vi "Check Mode.vi"(8 "error in (no error)":errorcluster, 11 "RT Data in in":T1 {"Channels"."Voltage"."Ref"."Data Reference" format="%.0x"; "Channels"."Current"."Ref"."Data Reference" format="%.0x"; "Channels"."Read Volt"."Ref" format="%.0x"; "Channels"."Mode"."Ref" format="%.0x"}) -> (0 "error out":errorcluster, 3 "RT Data out":T1 {"Channels"."Voltage"."Ref"."Data Reference" format="%.0x"; "Channels"."Current"."Ref"."Data Reference" format="%.0x"; "Channels"."Read Volt"."Ref" format="%.0x"; "Channels"."Mode"."Ref" format="%.0x"})   [LabVIEW 2011, in "Switch-DMM Custom Device.lvlib"]
uses:
  Switch-DMM Custom Device.lvlib
  Controls/RT Data.ctl
  Controls/Channels.ctl
  Controls/Single Channel.ctl
  <vilib>/NI Veristand/Custom Device API/Data Reference.ctl
  Controls/Block Channels.ctl
  <vilib>/NI Veristand/Custom Device API/Block Data Reference.ctl
  Controls/Communication.ctl
  Controls/Async Status.ctl
  Controls/Async State.ctl
  Controls/Async Command.ctl
  Controls/Async Events.ctl
  <vilib>/NI Veristand/Custom Device API/Global Data Refs.vi
  <vilib>/NI Veristand/Custom Device API/Custom Device API.lvlib
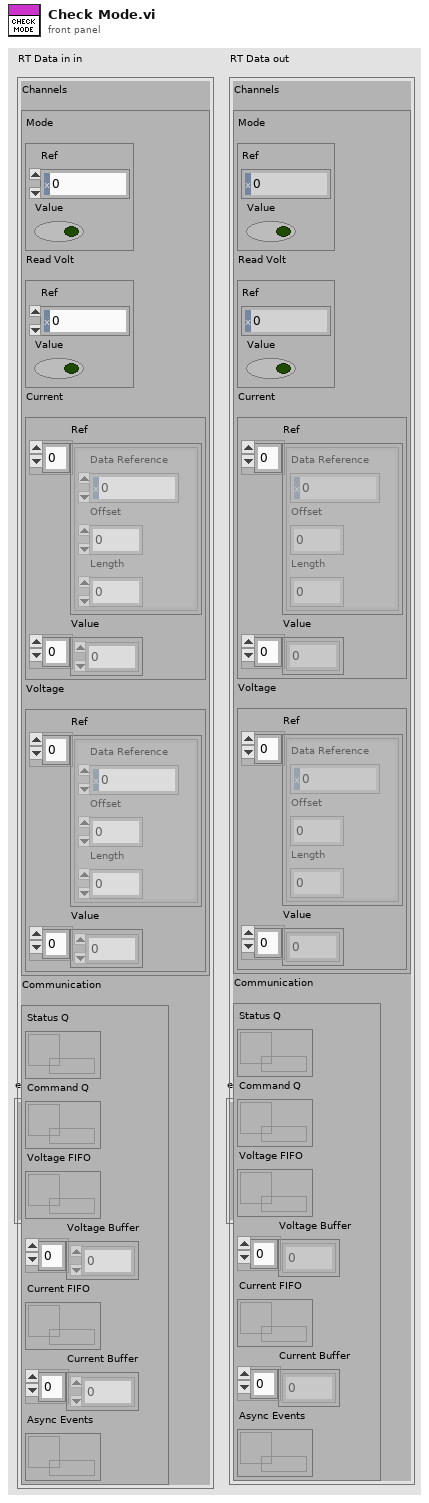
[diagram p1: front panel]
types:
  T1 = typedef "Switch-DMM Custom Device.lvlib/RT Data.ctl" = cluster{"Channels":T2, "Communication":T7}
  T2 = typedef "Switch-DMM Custom Device.lvlib/Channels.ctl" = cluster{"Mode":T3, "Read Volt":T3, "Current":T5, "Voltage":T5}
  T3 = typedef "Switch-DMM Custom Device.lvlib/Single Channel.ctl" = cluster{"Ref":T4, "Value":bool}
  T4 = typedef "Custom Device API.lvlib/Data Reference.ctl" = i32
  T5 = typedef "Switch-DMM Custom Device.lvlib/Block Channels.ctl" = cluster{"Ref":T6[], "Value":dbl[]}
  T6 = typedef "Custom Device API.lvlib/Block Data Reference.ctl" = cluster{"Data Reference":T4, "Offset":i32, "Length":i32}
  T7 = typedef "Switch-DMM Custom Device.lvlib/Communication.ctl" = cluster{"Status Q":refnum<queue>, "Command Q":refnum<queue>, "Voltage FIFO":refnum<k33>, "Voltage Buffer":dbl[], "Current FIFO":refnum<k33>, "Current Buffer":dbl[], "Async Events":refnum<queue>}
  T8 = typedef "Switch-DMM Custom Device.lvlib/Async Command.ctl" = enum16{"None", "Start", "Set Cur Mode", "Req Volt Mode", "Set Volt Mode", "Read Volt", "Exit"}
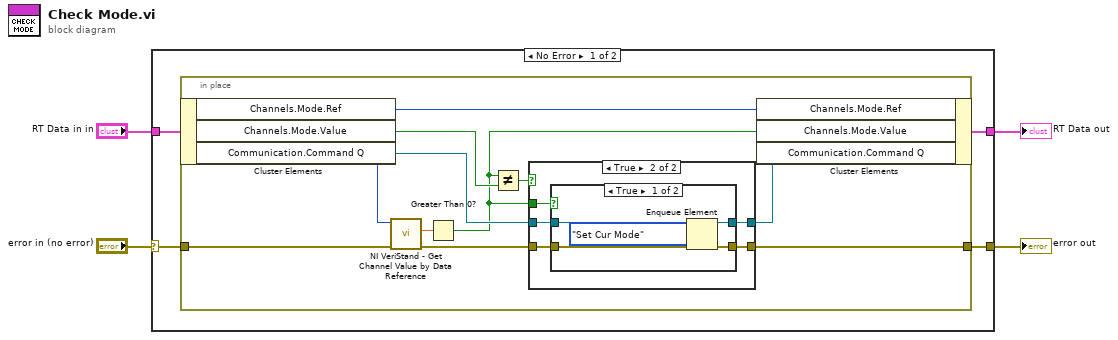
[diagram p0: block diagram]
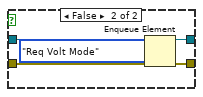
[diagram p3: hidden frame]
diagram:
  n1 = case shown="No Error" "error in (no error)" {
    selector: "error in (no error)" -> [w8 w36]
    tunnel: "RT Data in in" -> [w7 w37]
    tunnel: [w6 w37] -> w3
    tunnel: [w5 w36] -> w4
    frame No Error {
      n2 = in-place {
        in-place-border: w8 -> [w17]
        in-place-border: [w10] -> w5
        n3 = in-place-cluster #1(w7) -> ("Channels.Mode.Ref"=w18:T4, "Channels.Mode.Value"=w16:bool, "Communication.Command Q"=w13:refnum<queue>)
        n4 = call <vilib>:"NI VeriStand - Get Channel Value by Data Reference.vi"("error in (no error)"=w17, "Data Reference in"=w18) -> ("error out"=w11:errorcluster, "Value"=w14:dbl)  [unwired: 8 in]
        n5 = Greater Than 0?(x=w14) -> (x > 0?=w9:bool)
        n6 = Not Equal?(x=w9, y=w16) -> (x != y?=w15:bool)
        n7 = case shown="True" w15 {
          tunnel: w13 -> [w20 w24]
          tunnel: w9 -> [_ w25]
          tunnel: [w20 w23] -> w12
          tunnel: w11 -> [w19 w22]
          tunnel: [w19 w21] -> w10
          frame False {
          }
          frame True {
            n8 = case shown="True" w25 {
              tunnel: w24 -> [w30 w35]
              tunnel: [w29 w34] -> w23
              tunnel: w22 -> [w28 w33]
              tunnel: [w26 w31] -> w21
              frame True {
                n9 = Enqueue Element(queue=w30, element=Async_Command."Set Cur Mode", error in (no error)=w28) -> (queue out=w29:refnum<queue>, error out=w26:errorcluster)  [unwired: 1 in, 1 out]
              }
              frame False {
                n10 = Enqueue Element(queue=w35, element=Async_Command."Req Volt Mode", error in (no error)=w33) -> (queue out=w34:refnum<queue>, error out=w31:errorcluster)  [unwired: 1 in, 1 out]
              }
            }
          }
        }
        n11 = in-place-cluster #1("Channels.Mode.Ref"=w18, "Channels.Mode.Value"=w9, "Communication.Command Q"=w12) -> (w6:T1)
      }
    }
    frame Error {
    }
  }
  "error out" <- w4
  "RT Data out" <- w3
